vi "download file.vi"(8 "error in (no error)":errorcluster, 10 "timeout (10000)":i32=300000, 11 "远端地址":string="/updatefiles/OneStation/V4/一体化微型水质监测站.zip") -> (0 "error out":errorcluster, 3 "appended path":path)   [LabVIEW 2016, in "数据传输系统-02.lvlib" / "update.lvlib" / "http client.lvclass"]
uses:
  http client class/http client.lvclass
  http client class/http client.lvclass/http client.ctl
  update.lvlib
panel:
  out "通知":cluster{"文件大小":i64, "已下载大小":i64, "滑动杆":dbl}
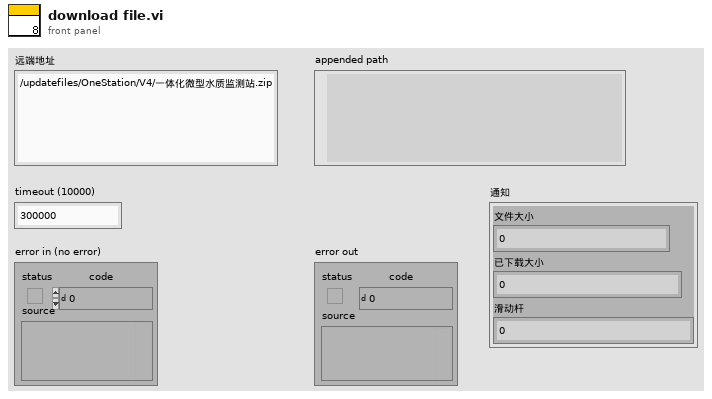
[diagram p1: front panel]
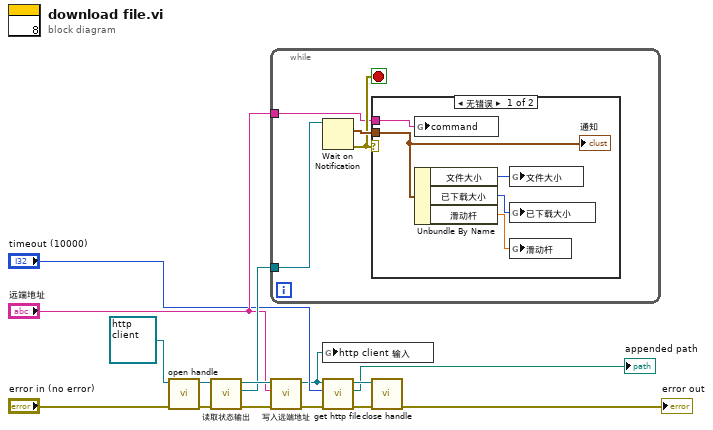
[diagram p0: block diagram]
diagram:
  n1 = call "open handle.vi"("error in (no error)"="error in (no error)", "http client 输入"=refnum<class "http client.lvclass"> refnum ("update.lvlib:http client.lvclass")) -> ("error out"=w11:errorcluster, "http client 输出"=w12:refnum<class "http client.lvclass">)  [unwired: 8 in]
  n2 = call "读取状态输出.vi"("error in (no error)"=w11, "http client输入"=w12) -> ("error out"=w9:errorcluster, "状态输出"=w8:refnum<notifier>, "http client输出"=w10:refnum<class "http client.lvclass">)  [unwired: 7 in]
  n3 = while {
    tunnel: w8 -> [w19]
    tunnel: "远端地址" -> [w16]
    stop <- w17 stop-if-true
    n4 = Wait on Notification(notifier=w19) -> (notification=w18:cluster{"文件大小":i64, "已下载大小":i64, "滑动杆":dbl}, error out=w17:errorcluster)  [unwired: 3 in, 2 out]
    n5 = case shown="无错误" w17 {
      tunnel: w18 -> [w24 _]
      tunnel: w16 -> [w20 _]
      frame No Error {
        n6 = global write "更新全局变量.vi" "command"(w20) -> ()
        n7 = Unbundle By Name(w24) -> ("文件大小"=w21:i64, "已下载大小"=w23:i64, "滑动杆"=w22:dbl)
        n8 = global write "更新全局变量.vi" "文件大小"(w21) -> ()
        n9 = global write "更新全局变量.vi" "已下载大小"(w23) -> ()
        n10 = global write "更新全局变量.vi" "滑动杆"(w22) -> ()
        "通知" <- w24
      }
      frame Error {
      }
    }
  }
  n11 = call "写入远端地址.vi"("error in (no error)"=w9, "远端地址"="远端地址", "http client输入"=w10) -> ("error out"=w15:errorcluster, "http client输出"=w4:refnum<class "http client.lvclass">)  [unwired: 7 in]
  n12 = global write "更新全局变量.vi" "http client 输入"(w4) -> ()
  n13 = call "get http file.vi"("error in (no error)"=w15, "timeout (10000)"="timeout (10000)", "http client 输入"=w4) -> ("error out"=w13:errorcluster, "appended path"=→"appended path":path, "http client 输出"=w14:refnum<class "http client.lvclass">)  [unwired: 6 in]
  n14 = call "close handle.vi"("error in (no error)"=w13, "http client 输入"=w14) -> ("error out"=→"error out":errorcluster)  [unwired: 8 in, 1 out]
